vi "Upload Segment.vi"(11 "Service Data Object in":refnum<class "Service Data Object.lvclass">) -> (1 "Request":refnum<class "CANopen Request Message.lvclass">, 2 "Expected Response":refnum<class "CANopen Response Message.lvclass">, 3 "Service Data Object out":refnum<class "Service Data Object.lvclass">)   [LabVIEW 2024, in "Service Data Object.lvclass"]
uses:
  Service Data Object.lvclass
  Service Data Object.lvclass/Service Data Object.ctl
  Upload Segment Response Comparator/Upload Segment Response Comparator.lvclass
  CANopen Request/CANopen Request Message.lvclass
  CANopen Message/CANopen Message.lvclass
  source/Typedefs/Function Code.ctl
  source/CANopen.lvlib
  SDO Response Compare Strategy/SDO Response Compare Strategy.lvclass
  e98d613c-e21d-48f3-9845-2be285cbd5d0.vi
  CANopen Response/CANopen Response Message.lvclass
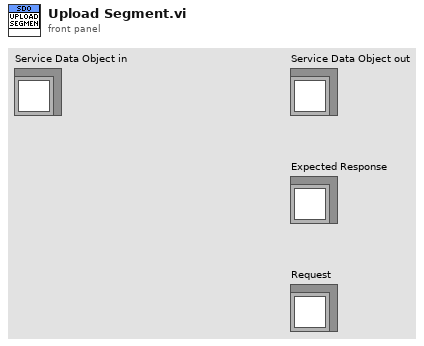
[diagram p1: front panel]
types:
  T1 = typedef "CANopen.lvlib/Function Code.ctl" = u8
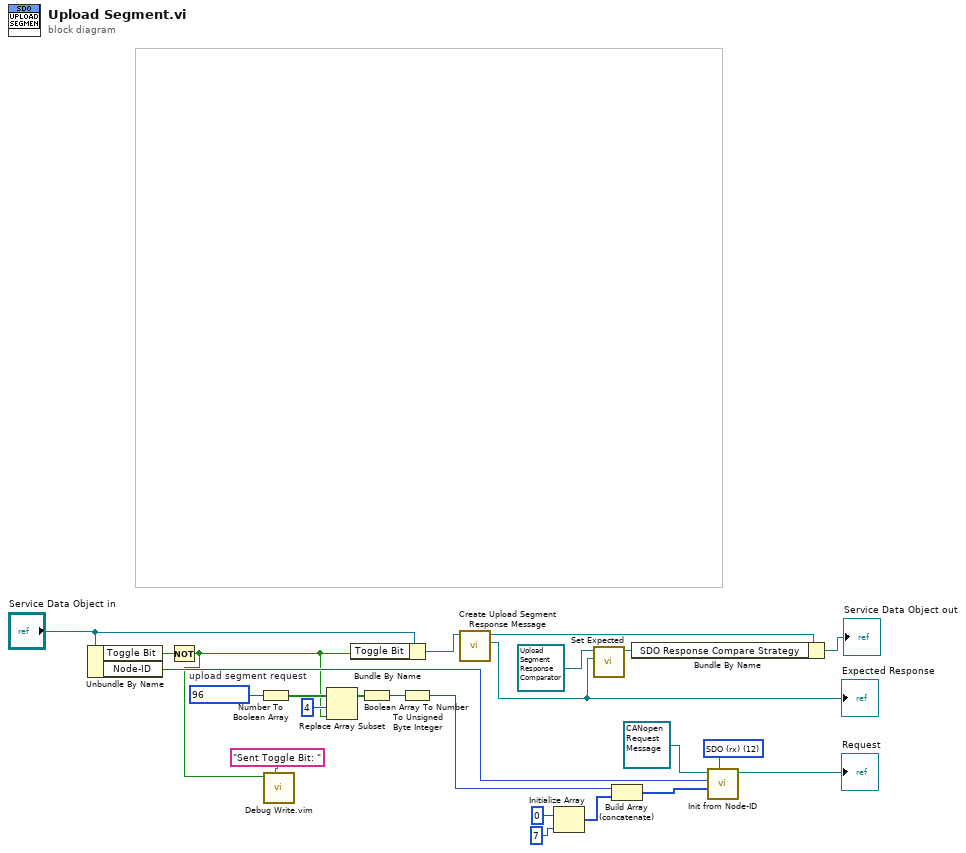
[diagram p0: block diagram]
diagram:
  w24 = T1 12 items=["NMT"=0, "EMCY/SYNC"=1, "TIME"=2, "PDO1 (tx)"=3, "PDO1 (rx)"=4, "PDO2 (tx)"=5, "PDO2 (rx)"=6, "PDO3 (tx)"=7, "PDO3 (rx)"=8, "PDO4 (tx)"=9, "PDO4 (rx)"=10, "SDO (tx)"=11, "SDO (rx)"=12, "NMT error control"=14] ("Function code")
  w18 = u8 96  # upload segment request
  n1 = Unbundle By Name("Service Data Object in") -> ("Toggle Bit"=w19:bool, "Node-ID"=w6:u8)
  n2 = Not(x=w19) -> (.not. x?=w1:bool)
  n3 = Number To Boolean Array(number=w18) -> (Boolean array=w17:bool[])
  n4 = call "Debug Write.vim"("prefix (\"\")"="Sent Toggle Bit: " ("prefix (\"\")"), "value"=w1) -> ()  [unwired: 9 in, 1 out]
  n5 = Replace Array Subset(array=w17, new element=w1, index=4) -> (w15:bool[])
  n6 = Bundle By Name(cluster="Service Data Object in", "Toggle Bit"=w1) -> (w20:refnum<class "Service Data Object.lvclass">)
  n7 = Boolean Array To Number(Boolean array=w15) -> (number=w14:u32)
  n8 = To Unsigned Byte Integer(number=w14) -> (unsigned 8bit integer=w13:u8)
  n9 = call "Create Upload Segment Response Message.vi"("Service Data Object in"=w20) -> ("Response Message"=w10:refnum<class "CANopen Response Message.lvclass">, "Service Data Object out"=w12:refnum<class "Service Data Object.lvclass">)  [unwired: 9 in]
  "Expected Response" <- w10
  n10 = Initialize Array(u8 0, 7 ("y")) -> (w3:u8[])
  n11 = call "Set Expected.vi"("CANopen Message"=w10, "SDO Response Compare Strategy in"=refnum<class "Upload Segment Response Comparator.lvclass"> refnum ("CANopen Master.lvlib:Upload Segment Response Comparator")) -> ("SDO Response Compare Strategy out"=w9:refnum<class "Upload Segment Response Comparator.lvclass">)  [unwired: 9 in]
  n12 = Build Array (concatenate)(w13, w3) -> (w23:u8[])
  n13 = Bundle By Name(cluster=w12, "SDO Response Compare Strategy"=w9) -> (→"Service Data Object out":refnum<class "Service Data Object.lvclass">)
  n14 = call "Init from Node-ID.vi"("Function Code"=w24, "Data"=w23, "Node-ID"=w6, 11:refnum<class "CANopen Request Message.lvclass"> refnum ("CANopen Master.lvlib:CANopen Request Message.lvclass")) -> ("CANopen Message"=→"Request":refnum<class "CANopen Message.lvclass">)  [unwired: 7 in]
